vi "EMV T7 Flow Detect.vi"(4 "Abnormal Input Temperature":dbl=90.0, 6 "T7_DELTA_INDICATING_FLOW":dbl, 8 "error in (no error)":errorcluster, 9 "Cold Water Supply Temperature":dbl, 10 "T7_DELTA_FLOW_THRESHOLD":dbl, 11 "T7 Temp":dbl=140.0) -> (0 "error out":errorcluster, 1 "Slope Chart 2":dbl(graph), 2 "Current T7 Temperatures":dbl[](array[numeric]), 3 "T7 Detect?":bool)   [LabVIEW 2016]
panel:
  out "Slope of Slope Chart":dbl(graph)
  out "slope of slope":dbl
  out "slope standard deviation":dbl format="%0.2f"
  out "Slope History":dbl[](array[numeric])
  out "slope":dbl
  out "standard deviation":dbl format="%0.2f"
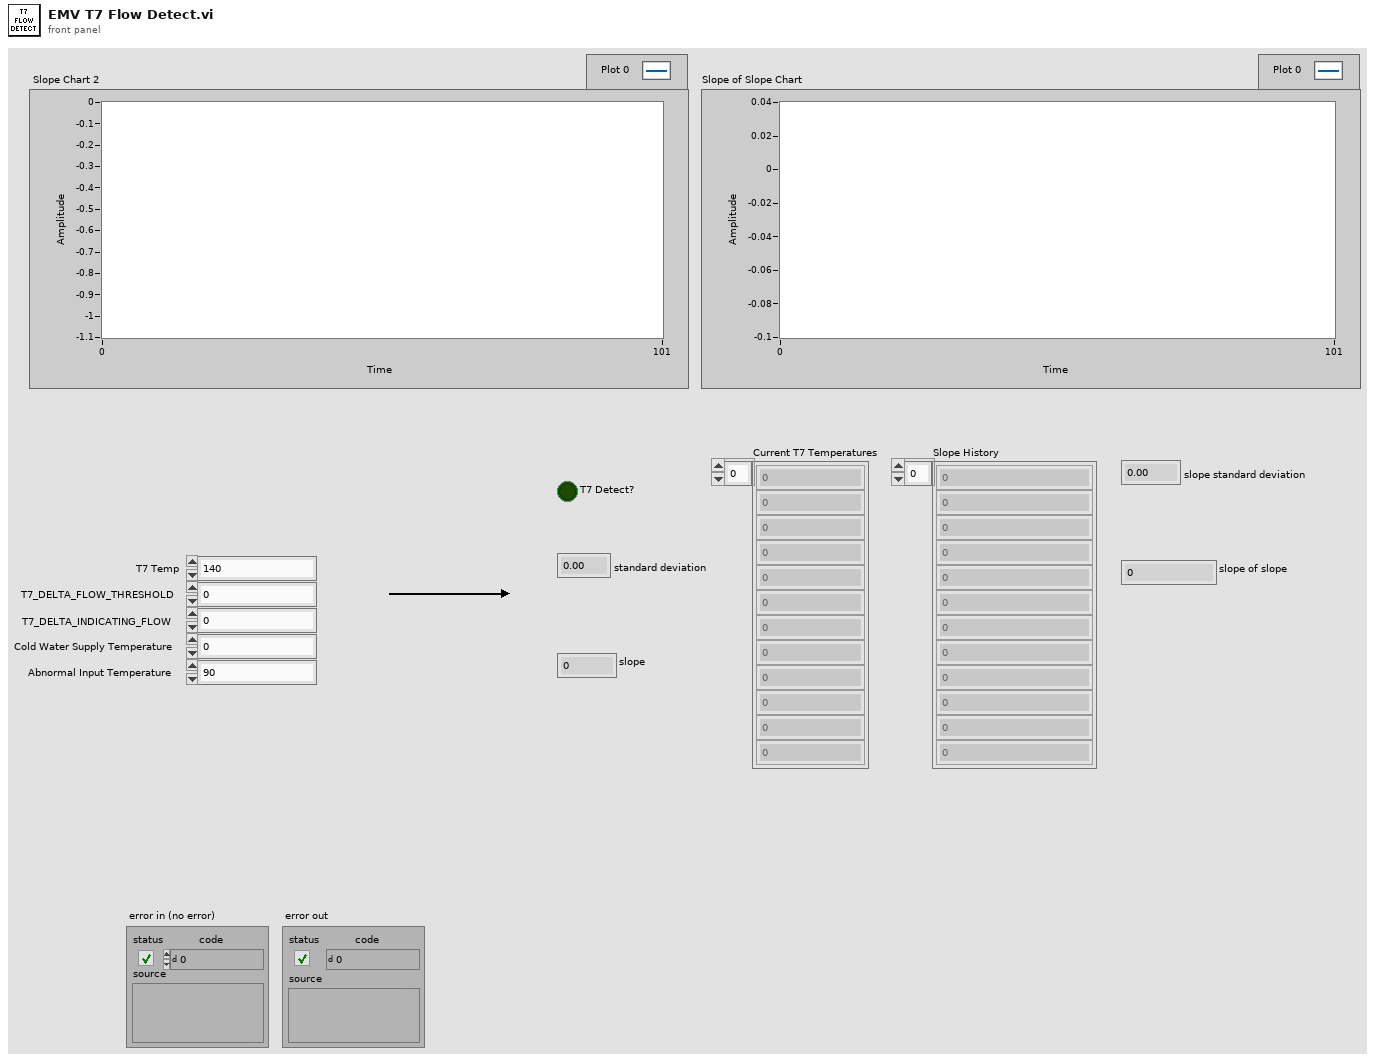
[diagram p1: front panel]
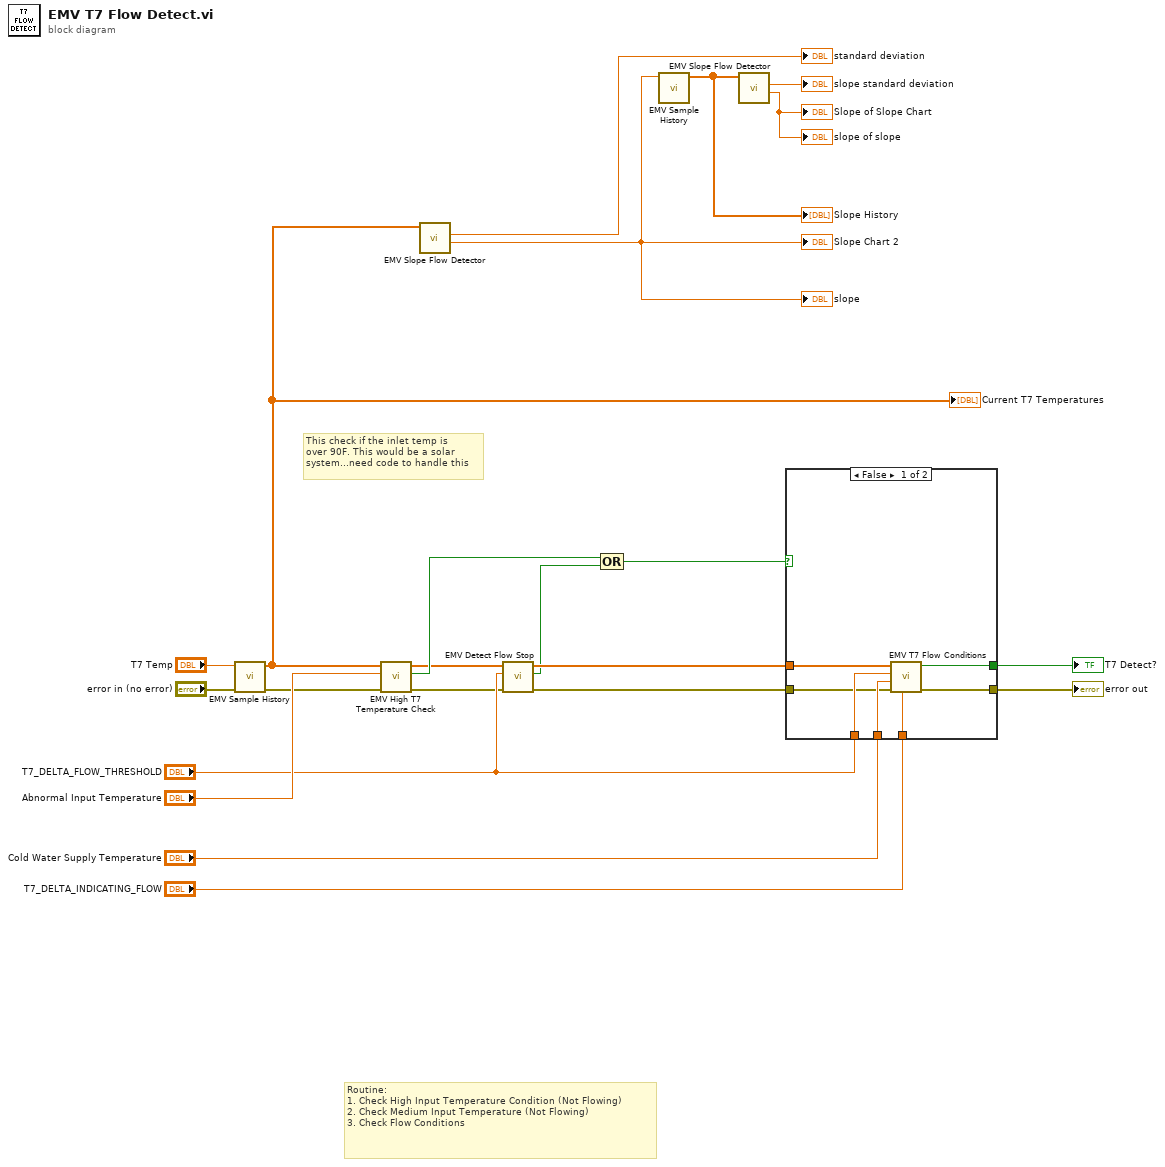
[diagram p0: block diagram]
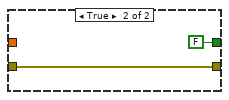
[diagram p2: hidden frame]
diagram:
  # "This check if the inlet temp is \nover 90F. This would be a solar \nsystem...need code to handle this"
  # "Routine:\n1. Check High Input Temperature Condition (Not Flowing)\n2. Check Medium Input Temperature (Not Flowing)\n3. Check Flow Conditions"
  n1 = call "EMV Sample History.vi"("error in (no error)"="error in (no error)", "T6 Temp"="T7 Temp") -> ("error out"=w11:errorcluster, "T6 History"=w13:dbl[])  [unwired: 8 in]
  "Current T7 Temperatures" <- w13
  n2 = call "EMV High T7 Temperature Check.vi"("error in (no error)"=w11, "Abnormal Input Temperature"="Abnormal Input Temperature", "T6 History"=w13) -> ("error out"=w4:errorcluster, "Hot Inlet Water?"=w8:bool, "T6 History Output"=w6:dbl[])  [unwired: 6 in]
  n3 = call "EMV Slope Flow Detector.vi"("Current T6 Temperatures in"=w13) -> ("slope"=w15:dbl, "standard deviation"=→"standard deviation":dbl)  [unwired: 6 in, 3 out]
  "slope" <- w15
  "Slope Chart 2" <- w15
  n4 = call "EMV Detect Flow Stop.vi"("error in (no error)"=w4, "T7_DELTA_FLOW_THRESHOLD"="T7_DELTA_FLOW_THRESHOLD", "T6 History Output"=w6) -> ("error out"=w3:errorcluster, "Detection"=w1:bool, "Current T7 Temperatures Output"=w2:dbl[])  [unwired: 6 in]
  n5 = Compound Arithmetic op=OR(w8, w1) -> (w7:bool)
  n6 = call "EMV Sample History.vi"("T6 Temp"=w15) -> ("T6 History"=w18:dbl[])  [unwired: 9 in, 1 out]
  "Slope History" <- w18
  n7 = call "EMV Slope Flow Detector.vi"("Current T6 Temperatures in"=w18) -> ("slope"=→"slope of slope" →"Slope of Slope Chart":dbl, "standard deviation"=→"slope standard deviation":dbl)  [unwired: 6 in, 3 out]
  n8 = case shown="False" w7 {
    tunnel: "Cold Water Supply Temperature" -> [w29 _]
    tunnel: [w28 FALSE ("T7 Detect?")] -> w17
    tunnel: [w27 w30] -> w16
    tunnel: "T7_DELTA_INDICATING_FLOW" -> [w26 _]
    tunnel: "T7_DELTA_FLOW_THRESHOLD" -> [w25 _]
    tunnel: w3 -> [w24 w30]
    tunnel: w2 -> [w23 _]
    frame False {
      n9 = call "EMV T7 Flow Conditions.vi"("T7_DELTA_INDICATING_FLOW"=w26, "error in (no error)"=w24, "Cold Water Supply Temperature"=w29, "T7_DELTA_FLOW_THRESHOLD"=w25, "T7 History"=w23) -> ("error out"=w27:errorcluster, "T7 Detect?"=w28:bool)  [unwired: 5 in]
    }
    frame True {
    }
  }
  "T7 Detect?" <- w17
  "error out" <- w16
